vi "test13-LocalExternalStateRegistrationViaAPI.vi"(8 "error in (no error)":errorcluster, 11 "TestCase in":refnum<class "testcase-CSMBroadcast.lvclass">) -> (0 "error out":errorcluster, 3 "TestCase out":refnum<class "testcase-CSMBroadcast.lvclass">)   [LabVIEW 2017, in "testcase-CSMBroadcast.lvclass"]
uses:
  testcase-CSMBroadcast.lvclass
  0b17d103-e67b-41be-a9eb-a2ee1311ff1f.vi
  5999693e-4f8a-4b34-ae87-f34dff5771be.vi
  52a2a10a-a04b-4bad-8df4-e1eb944f47cc.vi
  826f03dd-b4b5-4c6b-9085-8edf6da4f43b.vi
  src/user.lib/_NEVSTOP/Communicable State Machine(CSM)/AdvanceAPI/CSM - Get Module Attribute.vi
  <vilib>/addons/_JKI Toolkits/VI Tester/TestCase.llb/TestCase.lvclass
  src/user.lib/_NEVSTOP/Communicable State Machine(CSM)/Communicable State Machine.lvlib
  CSM/CSM-Testcase.lvlib
  C:/Program Files (x86)/National Instruments/LabVIEW 2017/vi.lib/addons/_JKI Toolkits/VI Tester/TestCase.llb/TestCase.lvclass
panel:
  out "LoopCount 2":i32
  out "LoopCount":i32
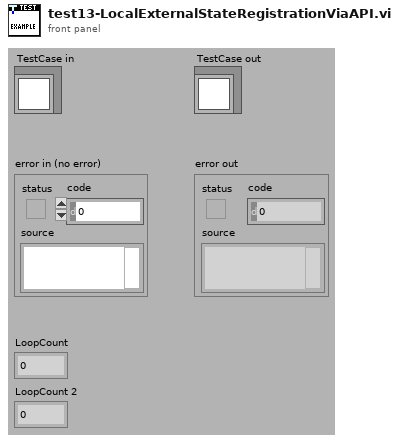
[diagram p1: front panel]
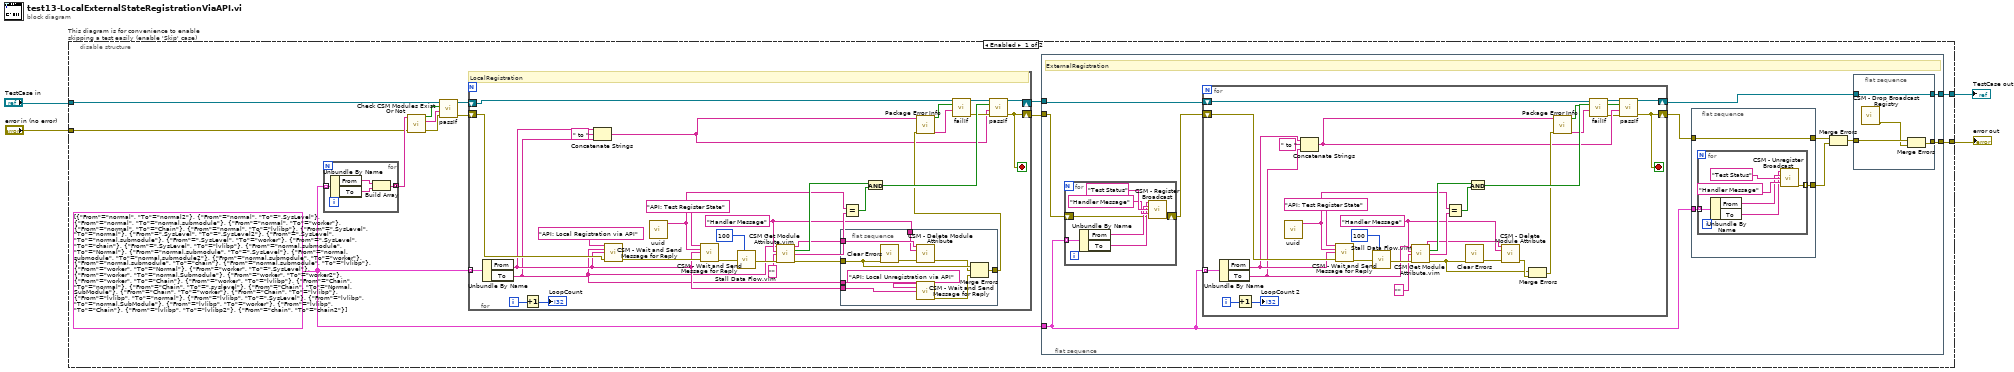
[diagram p0: block diagram]
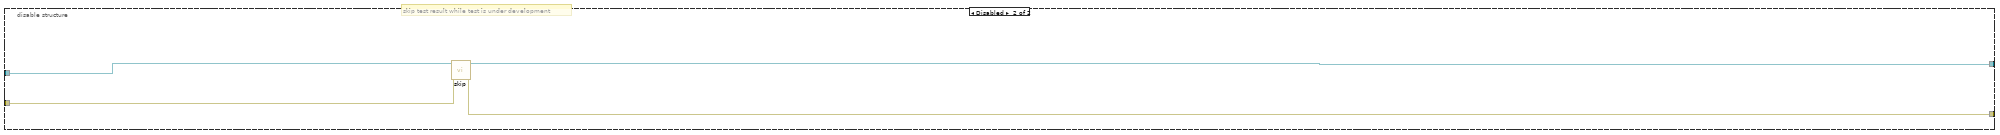
[diagram p2: hidden frame]
diagram:
  n1 = disable-structure "This diagram is for convenience to enable skipping a test easily (enable 'Skip' case)" shown="Enabled" {
    disable-tunnel: "TestCase in" -> [w7 w128]
    disable-tunnel: [w16 w126] -> w1
    disable-tunnel: [w14 w127] -> w3
    disable-tunnel: "error in (no error)" -> [w6 w125]
    frame Enabled {
      w5 = cluster{"From":string, "To":string}[] [{"From"="normal", "To"="normal2"}, {"From"="normal", "To"=".SysLevel"}, {"From"="normal", "To"="normal.submodule"}, {"From"="normal", "To"="worker"}, {"From"="normal", "To"="Chain"}, {"From"="normal", "To"="lvlibp"}, {"From"=".SysLevel", "To"="normal"}, {"From"=".SysLevel", "To"=".SysLevel2"}, {"From"=".SysLevel", "To"="normal.submodule"}, {"From"=".SysLevel", "To"="worker"}, {"From"=".SysLevel", "To"="chain"}, {"From"=".SysLevel", "To"="lvlibp"}, {"From"="normal.submodule", "To"="Normal"}, {"From"="normal.submodule", "To"=".SysLevel"}, {"From"="normal.submodule", "To"="normal.submodule2"}, {"From"="normal.submodule", "To"="worker"}, {"From"="normal.submodule", "To"="chain"}, {"From"="normal.submodule", "To"="lvlibp"}, {"From"="worker", "To"="Normal"}, {"From"="worker", "To"=".SysLevel"}, {"From"="worker", "To"="normal.Submodule"}, {"From"="worker", "To"="worker2"}, {"From"="worker", "To"="Chain"}, {"From"="worker", "To"="lvlibp"}, {"From"="Chain", "To"="normal"}, {"From"="Chain", "To"=".syslevel"}, {"From"="Chain", "To"="Normal.SubModule"}, {"From"="Chain", "To"="worker"}, {"From"="Chain", "To"="lvlibp"}, {"From"="lvlibp", "To"="normal"}, {"From"="lvlibp", "To"=".SysLevel"}, {"From"="lvlibp", "To"="normal.SubModule"}, {"From"="lvlibp", "To"="worker"}, {"From"="lvlibp", "To"="Chain"}, {"From"="lvlibp", "To"="lvlibp2"}, {"From"="chain", "To"="chain2"}]
      n2 = for {
        tunnel: w5 -> [w21] mode=indexing
        tunnel: [w18] -> w12 mode=concatenating
        n3 = Unbundle By Name(w21) -> ("From"=w20:string, "To"=w19:string)
        n4 = Build Array(w20, w19) -> (w18:string[])
      }
      n5 = call "Check CSM Modules Exist Or Not.vi"("error in"=w6, "CSM names in"=w12) -> ("error out"=w10:errorcluster, "Debug string"=w11:string, "All Modules Exist?"=w13:bool)  [unwired: 7 in]
      n6 = call-dynamic "passIf.vi"("error in (no error)"=w10, "message (\"\")"=w11, "pass"=w13, "TestCase in"=w7) -> ("error out"=w9:errorcluster, "TestCase out"=w8:refnum<class "testcase-CSMBroadcast.lvclass">)  [unwired: 6 in]
      n7 = for {
        shift-right: [w32] -> w15
        shift-left: w9 -> [w33]
        shift-right: [w39] -> w17
        shift-left: w8 -> [w29]
        tunnel: w5 -> [w50] mode=indexing
        i -> [w52]
        stop <- w32 stop-if-true
        w34 = "Handler Message" ("To")
        # "LocalRegistration"
        n8 = Unbundle By Name(w50) -> ("From"=w25:string, "To"=w24:string)
        n9 = Increment(x=w52) -> (x+1=→"LoopCount":i32)
        n10 = Concatenate Strings(w25, " to " ("string"), w24) -> (w22:string)
        n11 = call "CSM - Wait and Send Message for Reply.vi"("State"="API: Local Registration via API", "Arguments (\"\")"=w24, "Target Module"=w25, "Error In (No Error)"=w33) -> ("error out"=w47:errorcluster)  [unwired: 8 in, 3 out]
        n12 = call "uuid.vi"() -> ("UUID"=w41:string)  [unwired: 11 in]
        n13 = call "CSM - Wait and Send Message for Reply.vi"("State"="API: Test Register State", "Arguments (\"\")"=w41, "Target Module"=w25, "Error In (No Error)"=w47) -> ("error out"=w46:errorcluster)  [unwired: 8 in, 3 out]
        n14 = call "Stall Data Flow.vim"("value in"=w46, "milliseconds to wait"=u32 100) -> ("value out"=w44:errorcluster)  [unwired: 1 out]
        n15 = call "CSM Get Module Attribute.vim"("CSM Name"=w24, "Attribute"=w34, "Default Value (Empty Variant)"="", "Error In"=w44) -> ("CSM Name (Dup)"=w35:string, "Found"=w43:bool, "Value"=w40:string, "error out"=w36:errorcluster)  [unwired: 7 in, 1 out]
        n16 = flat-sequence {
          tunnel: w36 -> [w56]
          tunnel: w35 -> [w61]
          tunnel: w34 -> [w60]
          tunnel: w24 -> [w58]
          tunnel: w25 -> [w57]
          tunnel: [w53] -> w26
          frame #0 {
            n17 = call <vilib>:"Clear Errors.vi"("error in (no error)"=w56) -> ("error out"=w62:errorcluster)  [unwired: 5 in, 1 out]
            n18 = call "CSM - Delete Module Attribute.vi"("CSM Name"=w61, "Attribute"=w60, "Error In"=w62) -> ("error out"=w55:errorcluster)  [unwired: 9 in, 3 out]
            n19 = call "CSM - Wait and Send Message for Reply.vi"("State"="API: Local Unregistration via API", "Arguments (\"\")"=w58, "Target Module"=w57) -> ("error out"=w54:errorcluster)  [unwired: 9 in, 3 out]
            n20 = Merge Errors(w56, w55, w54) -> (w53:errorcluster)
          }
        }
        n21 = Equal?(x=w41, y=w40) -> (x = y?=w38:bool)
        n22 = And(x=w43, y=w38) -> (x .and. y?=w37:bool)
        n23 = call "Package Error Info.vi"("error in"=w26, "String in"=w22) -> ("packed error info out"=w30:string, "error status"=w31:bool)  [unwired: 8 in]
        n24 = call-dynamic "failIf.vi"("message (\"\")"=w30, "fail"=w31, "TestCase in"=w29) -> ("error out"=w27:errorcluster, "TestCase out"=w28:refnum<class "testcase-CSMBroadcast.lvclass">)  [unwired: 7 in]
        n25 = call-dynamic "passIf.vi"("error in (no error)"=w27, "message (\"\")"=w22, "pass"=w37, "TestCase in"=w28) -> ("error out"=w32:errorcluster, "TestCase out"=w39:refnum<class "testcase-CSMBroadcast.lvclass">)  [unwired: 6 in]
      }
      n26 = flat-sequence {
        tunnel: w17 -> [w73]
        tunnel: [w67] -> w16
        tunnel: w15 -> [w64]
        tunnel: w5 -> [w72]
        tunnel: [w69] -> w14
        frame #0 {
          # "ExternalRegistration"
          n27 = for {
            tunnel: w72 -> [w93] mode=indexing
            shift-right: [w88] -> w63
            shift-left: w64 -> [w87]
            n28 = Unbundle By Name(w93) -> ("From"=w90:string, "To"=w89:string)
            n29 = call "CSM - Register Broadcast.vi"("CSM Name(Empty for Broadcast Event)"=w89, "Source CSM Name (* as Default)"=w90, "Trigger"="Test Status" ("Status"), "API (If \"\", Same as Trigger)"="Handler Message" ("Response Message (If \"\", Same as Source Message)"), "Error In"=w87) -> ("error out"=w88:errorcluster)  [unwired: 9 in, 1 out]
          }
          n30 = for {
            shift-right: [w107] -> w66
            shift-left: w63 -> [w106]
            shift-right: [w113] -> w68
            shift-left: w73 -> [w96]
            tunnel: w72 -> [w122] mode=indexing
            i -> [w124]
            stop <- w107 stop-if-true
            w108 = "Handler Message" ("To")
            n31 = Unbundle By Name(w122) -> ("From"=w99:string, "To"=w98:string)
            n32 = Increment(x=w124) -> (x+1=→"LoopCount 2":i32)
            n33 = call "uuid.vi"() -> ("UUID"=w115:string)  [unwired: 11 in]
            n34 = Concatenate Strings(w99, " to " ("string"), w98) -> (w97:string)
            n35 = call "CSM - Wait and Send Message for Reply.vi"("State"="API: Test Register State", "Arguments (\"\")"=w115, "Target Module"=w99, "Error In (No Error)"=w106) -> ("error out"=w120:errorcluster)  [unwired: 8 in, 3 out]
            n36 = call "Stall Data Flow.vim"("value in"=w120, "milliseconds to wait"=u32 100) -> ("value out"=w118:errorcluster)  [unwired: 1 out]
            n37 = call "CSM Get Module Attribute.vim"("CSM Name"=w98, "Attribute"=w108, "Default Value (Empty Variant)"="", "Error In"=w118) -> ("CSM Name (Dup)"=w109:string, "Found"=w117:bool, "Value"=w114:string, "error out"=w104:errorcluster)  [unwired: 7 in, 1 out]
            n38 = Equal?(x=w115, y=w114) -> (x = y?=w112:bool)
            n39 = call <vilib>:"Clear Errors.vi"("error in (no error)"=w104) -> ("error out"=w110:errorcluster)  [unwired: 5 in, 1 out]
            n40 = And(x=w117, y=w112) -> (x .and. y?=w111:bool)
            n41 = call "CSM - Delete Module Attribute.vi"("CSM Name"=w109, "Attribute"=w108, "Error In"=w110) -> ("error out"=w105:errorcluster)  [unwired: 9 in, 3 out]
            n42 = Merge Errors(w104, w105) -> (w101:errorcluster)
            n43 = call "Package Error Info.vi"("error in"=w101, "String in"=w97) -> ("packed error info out"=w102:string, "error status"=w103:bool)  [unwired: 8 in]
            n44 = call-dynamic "failIf.vi"("message (\"\")"=w102, "fail"=w103, "TestCase in"=w96) -> ("error out"=w94:errorcluster, "TestCase out"=w95:refnum<class "testcase-CSMBroadcast.lvclass">)  [unwired: 7 in]
            n45 = call-dynamic "passIf.vi"("error in (no error)"=w94, "message (\"\")"=w97, "pass"=w111, "TestCase in"=w95) -> ("error out"=w107:errorcluster, "TestCase out"=w113:refnum<class "testcase-CSMBroadcast.lvclass">)  [unwired: 6 in]
          }
          n46 = flat-sequence {
            tunnel: w72 -> [w76]
            tunnel: [w75] -> w71
            tunnel: w66 -> [w74]
            tunnel: [w74] -> w65
            frame #0 {
              n47 = for {
                tunnel: w76 -> [w82] mode=indexing
                tunnel: [w77] -> w75 mode=indexing
                n48 = Unbundle By Name(w82) -> ("From"=w79:string, "To"=w78:string)
                n49 = call "CSM - Unregister Broadcast.vi"("CSM Name(Empty for Broadcast Event)"=w78, "Source CSM Name (* as Default)"=w79, "Trigger"="Test Status" ("Status"), "API (\"*\" as Default)"="Handler Message" ("Response Message (If \"\", Same as Source Message)")) -> ("error out"=w77:errorcluster)  [unwired: 10 in, 1 out]
              }
            }
          }
          n50 = Merge Errors(w65, w71) -> (w70:errorcluster)
          n51 = flat-sequence {
            tunnel: w70 -> [w86]
            tunnel: [w85] -> w69
            tunnel: [w84] -> w67
            tunnel: w68 -> [w84]
            frame #0 {
              n52 = call "CSM - Drop Broadcast Registry.vi"() -> ("error out"=w83:errorcluster)  [unwired: 15 in]
              n53 = Merge Errors(w86, w83) -> (w85:errorcluster)
            }
          }
        }
      }
    }
    frame Disabled {
      # "skip test result while test is under development"
      n54 = call <vilib>:"skip.vi"("error in (no error)"=w125, "TestCase in"=w128) -> ("error out"=w127:errorcluster, "TestCase out"=w126:refnum<class "testcase-CSMBroadcast.lvclass">)  [unwired: 8 in]
    }
  }
  "error out" <- w3
  "TestCase out" <- w1
